vi "Linear stainless25 Calculations.vi"(0 "Power":dbl, 3 "X1":dbl[](array[numeric]), 5 "T1":dbl[](array[numeric]), 11 "X3":dbl[](array[numeric]), 12 "T3":dbl[](array[numeric])) -> (16 "Ks":dbl, 17 "Ky":dbl, 20 "XY Graph":cluster{"Ramp Pattern":dbl[], dbl[]}[](graph))   [LabVIEW 2017]
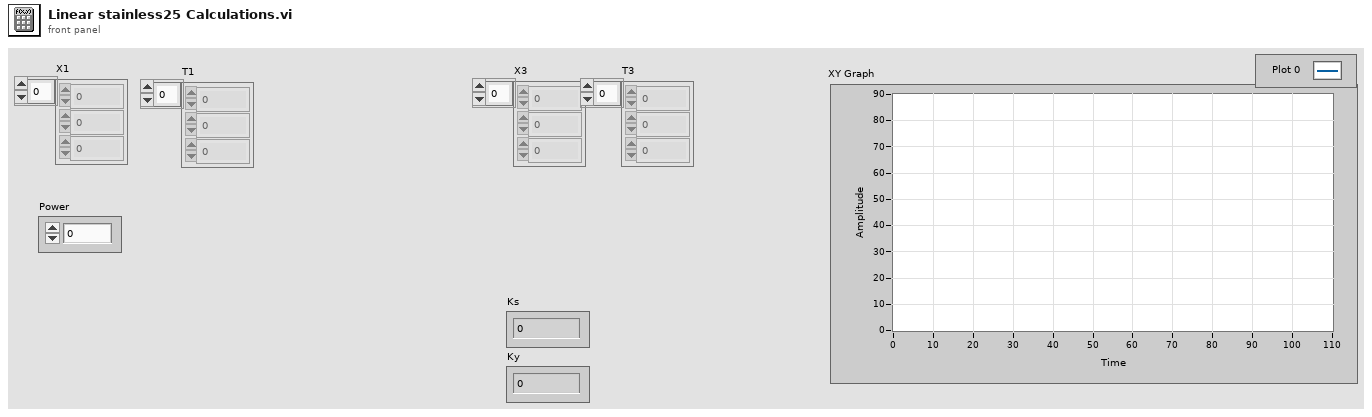
[diagram p1: front panel]
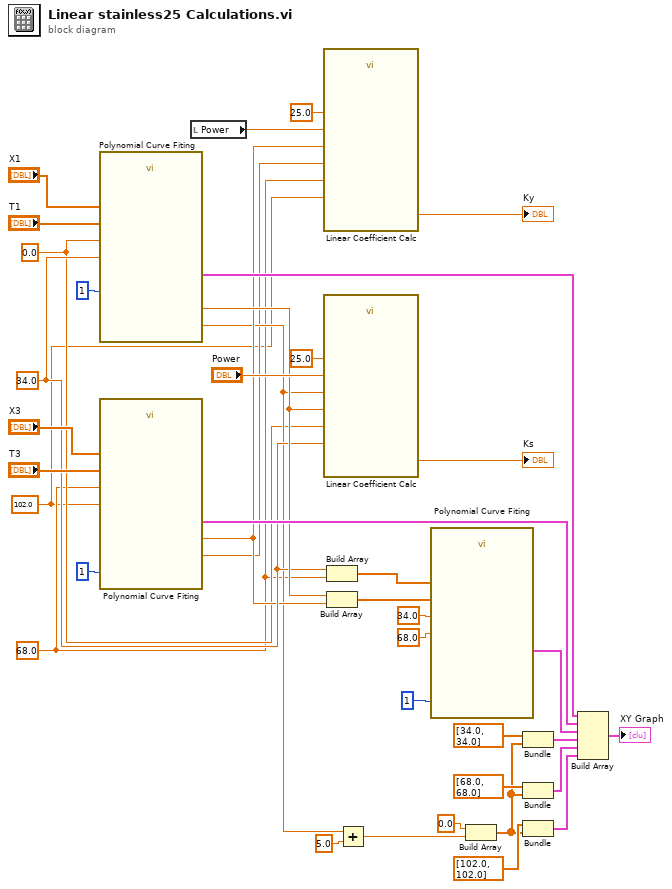
[diagram p0: block diagram]
diagram:
  w1 = 102.0 ("end")
  w2 = 68.0 ("start")
  w8 = 34.0 ("end")
  w4 = 0.0 ("start")
  n1 = call "Polynomial Curve Fiting.vi"("polynomial order"=1, "end"=w8, "start"=w4, "Y"="T1", "X"="X1") -> ("T Last"=w10:dbl, "T First"=w5:dbl, "XY Graph"=w32:cluster{"Ramp Pattern":dbl[], dbl[]})
  n2 = call "Polynomial Curve Fiting.vi"("polynomial order"=1, "end"=w1, "start"=w2, "Y"="T3", "X"="X3") -> ("T Last"=w3:dbl, "T First"=w6:dbl, "XY Graph"=w31:cluster{"Ramp Pattern":dbl[], dbl[]})
  n3 = local read "Power"() -> (w15:dbl)
  n4 = call "Linear Coefficient Calc.vi"("Diameter"=25.0, "Power"=w15, "X2"=w1, "X1"=w2, "T2"=w3, "T1"=w6) -> ("K"=→"Ky":dbl)
  n5 = call "Linear Coefficient Calc.vi"("Diameter"=25.0, "Power"="Power", "X2"=w8, "X1"=w4, "T2"=w10, "T1"=w5) -> ("K"=→"Ks":dbl)
  n6 = Build Array(w8, w2) -> (w12:dbl[])
  n7 = Build Array(w10, w6) -> (w11:dbl[])
  n8 = Add(x=w5, y=5.0) -> (x+y=w19:dbl)
  n9 = call "Polynomial Curve Fiting.vi"("polynomial order"=1, "end"=68.0, "start"=34.0, "Y"=w11, "X"=w12) -> ("XY Graph"=w30:cluster{"Ramp Pattern":dbl[], dbl[]})  [unwired: 2 out]
  n10 = Build Array(0.0 ("element"), w19) -> (w22:dbl[])
  n11 = Bundle("X Line 1"=dbl[] [34.0, 34.0], w22) -> (w26:cluster{"X Line 1":dbl[], dbl[]})  [unwired: 1 in]
  n12 = Bundle("X Line 2"=dbl[] [68.0, 68.0], w22) -> (w24:cluster{"X Line 2":dbl[], dbl[]})  [unwired: 1 in]
  n13 = Bundle("X Line 3"=dbl[] [102.0, 102.0], w22) -> (w21:cluster{"X Line 3":dbl[], dbl[]})  [unwired: 1 in]
  n14 = Build Array(w32, w31, w30, w26, w24, w21) -> (→"XY Graph":cluster{"X Line 3":dbl[], dbl[]}[])
